vi "DrawScatterPlot.vi"(0 "reference in":refnum<class "LcWebView.lvclass">, 2 "ScatterPlot.Dataset":cluster{"x":dbl, "y":dbl}[][](array[cluster]), 3 "Scatter.DatasetLabels":string[](array[string]), 5 "Error In":errorcluster, 6 "GenericPlotOptions":T2, 7 "ScatterPlot.PlotColours":u32[](array[numeric]), 8 "ScatterPlotOptions":T1={"xLabel"="", "yLabel"="", "DisplayXLabel"=TRUE, "DisplayYLabel"=TRUE}) -> (14 "reference out":refnum<class "LcWebView.lvclass">, 19 "Error Out":errorcluster)   [LabVIEW 2018, in "LcWebView.lvclass"]
uses:
  LcWebView.lvclass
  ctrls/GenericPlotOption.ctl
  ctrls/LegendPosition.ctl
  ctrls/LinePlotOption.ctl
  cdfa7b6c-348e-4618-b79e-b8b55caa0d01.vi
  <vilib>/JDP Science/JSONtext/Variant to JSON Text.vi
  <vilib>/JDP Science/JSONtext/LVClass Serializer/JSONtext LVClass Serializer.lvclass
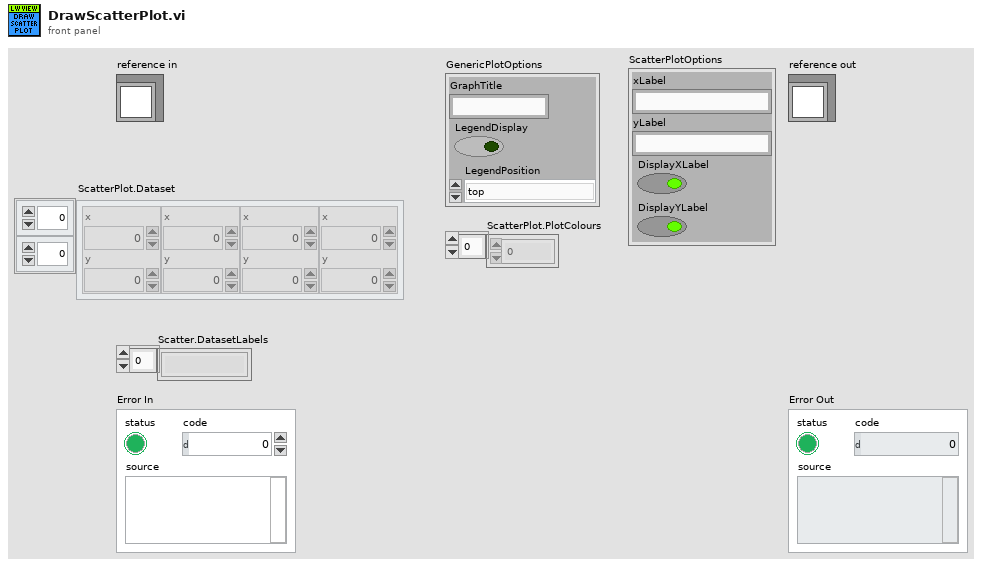
[diagram p1: front panel]
types:
  T1 = typedef "LcWebView.lvclass/LinePlotOption.ctl" = cluster{"xLabel":string, "yLabel":string, "DisplayXLabel":bool, "DisplayYLabel":bool}
  T2 = typedef "LcWebView.lvclass/GenericPlotOption.ctl" = cluster{"GraphTitle":string, "LegendDisplay":bool, "LegendPosition":T3}
  T3 = typedef "LcWebView.lvclass/LegendPosition.ctl" = enum16{"top", "right", "left", "bottom"}
  T4 = cluster{"action":string, "PlotData":string, "GenericPlotOptions":T2, "ScatterPlotOptions":T1}
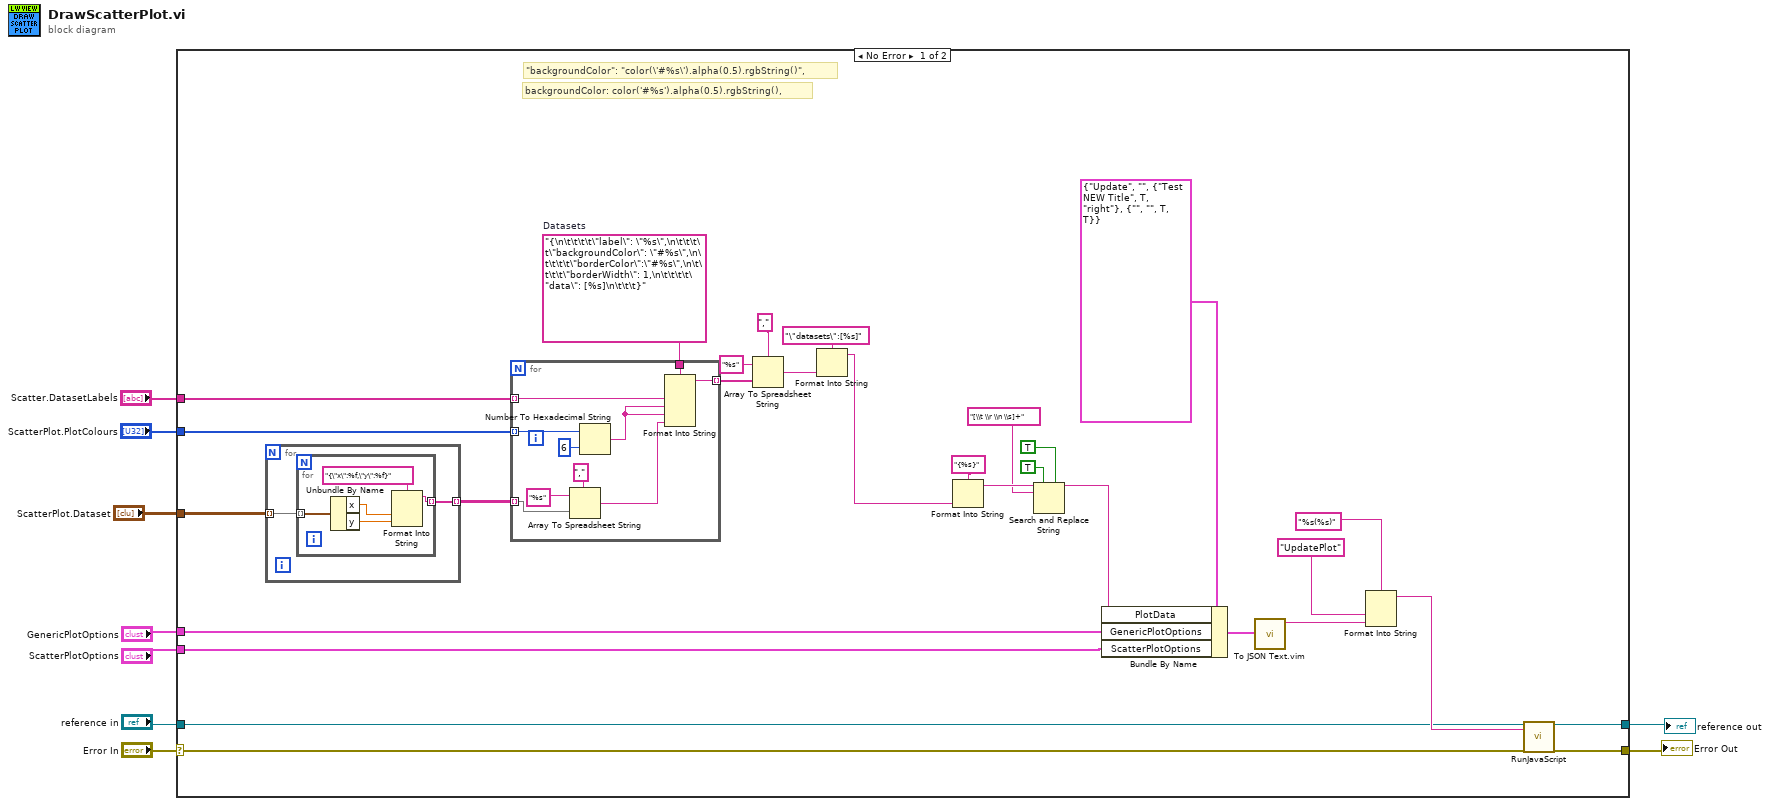
[diagram p0: block diagram]
diagram:
  n1 = case shown="No Error" "Error In" {
    selector: "Error In" -> [w17 w57]
    tunnel: [w18 w57] -> w2
    tunnel: [w19 w56] -> w3
    tunnel: "reference in" -> [w20 w56]
    tunnel: "ScatterPlot.Dataset" -> [w12 _]
    tunnel: "ScatterPlot.PlotColours" -> [w36 _]
    tunnel: "Scatter.DatasetLabels" -> [w35 _]
    tunnel: "GenericPlotOptions" -> [w28 _]
    tunnel: "ScatterPlotOptions" -> [w27 _]
    frame No Error {
      w37 = "{\n\t\t\t\t\"label\": \"%s\",\n\t\t\t\t\"backgroundColor\": \"#%s\",\n\t\t\t\t\"borderColor\":\"#%s\",\n\t\t\t\t\"borderWidth\": 1,\n\t\t\t\t\"data\": [%s]\n\t\t\t}"  # Datasets
      # "\"backgroundColor\": \"color(\\'#%s\\').alpha(0.5).rgbString()\","
      # "backgroundColor: color('#%s').alpha(0.5).rgbString(),"
      n2 = for {
        tunnel: w12 -> [w40] mode=indexing
        tunnel: [w39] -> w11 mode=indexing
        n3 = for {
          tunnel: w40 -> [w45] mode=indexing
          tunnel: [w41] -> w39 mode=indexing
          n4 = Unbundle By Name(w45) -> ("x"=w43:dbl, "y"=w42:dbl)
          n5 = Format Into String(format string="{\"x\":%f,\"y\":%f}", w43, w42) -> (resulting string=w41:string)  [unwired: 2 in, 1 out]
        }
      }
      n6 = for {
        tunnel: w36 -> [w52] mode=indexing
        tunnel: w35 -> [w54] mode=indexing
        tunnel: [w53] -> w16 mode=indexing
        tunnel: w37 -> [w55]
        tunnel: w11 -> [w49] mode=indexing
        n7 = Array To Spreadsheet String(delimiter (Tab)="," ("separator"), array=w49, 3:"%s" ("format string")) -> (spreadsheet string=w46:string)
        n8 = Number To Hexadecimal String(1:i16 6 ("width (-)"), 2:w52) -> (0:w51:string)
        n9 = Format Into String(format string=w55, w54, w51, w51, w46) -> (resulting string=w53:string)  [unwired: 2 in, 1 out]
      }
      n10 = Array To Spreadsheet String(delimiter (Tab)="," ("separator"), array=w16, 3:"%s" ("format string")) -> (spreadsheet string=w13:string)
      n11 = Format Into String(format string="\"datasets\":[%s]", w13) -> (resulting string=w10:string)  [unwired: 2 in, 1 out]
      n12 = Format Into String(format string="{%s}", w10) -> (resulting string=w33:string)  [unwired: 2 in, 1 out]
      n13 = Search and Replace String(replace all?=TRUE ("replace all? (F)"), multiline?=TRUE ("multiline? (F)"), input string=w33, search string="[\\t \\r \\n \\s]+") -> (result string=w32:string)  [unwired: 4 in, 3 out]
      n14 = Bundle By Name(cluster=T4 {"action"="Update", "PlotData"="", "GenericPlotOptions"={"GraphTitle"="Test NEW Title", "LegendDisplay"=TRUE, "LegendPosition"=enum."right"}, "ScatterPlotOptions"={"xLabel"="", "yLabel"="", "DisplayXLabel"=TRUE, "DisplayYLabel"=TRUE}}, "PlotData"=w32, "GenericPlotOptions"=w28, "ScatterPlotOptions"=w27) -> (w25:T4)
      n15 = call "To JSON Text.vim"("Anything"=w25) -> ("<JSON>"=w22:string)  [unwired: 9 in, 1 out]
      n16 = Format Into String(format string="%s(%s)", "UpdatePlot" ("input 1"), w22) -> (resulting string=w21:string)  [unwired: 2 in, 1 out]
      n17 = call-dynamic "RunJavaScript.vi"("reference in"=w20, "Java Script Function"=w21, "Error In"=w17) -> ("reference out"=w19:refnum<class "LcWebView.lvclass">, "Error Out"=w18:errorcluster)  [unwired: 13 in, 2 out]
    }
    frame Error {
    }
  }
  "Error Out" <- w2
  "reference out" <- w3
